vi "lin-log.vi"(4 "W In 1":dbl, 5 "W In 2":dbl, 6 "W In 3":dbl, 7 "W In 4":dbl) -> (0 "dBm Out 1":dbl, 1 "dBm Out 2":dbl, 2 "dBm Out 3":dbl, 3 "dBm Out 4":dbl)   [LabVIEW 2015]
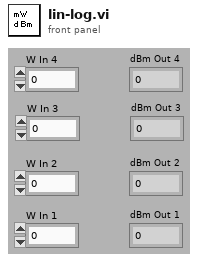
[diagram p1: front panel]
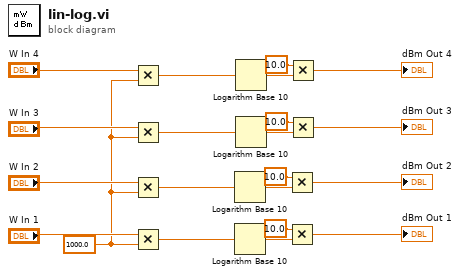
[diagram p0: block diagram]
diagram:
  w1 = 1000.0 ("y")
  n1 = Multiply(x="W In 4", y=w1) -> (x*y=w6:dbl)
  n2 = Multiply(x="W In 3", y=w1) -> (x*y=w7:dbl)
  n3 = Multiply(x="W In 2", y=w1) -> (x*y=w8:dbl)
  n4 = Multiply(x="W In 1", y=w1) -> (x*y=w9:dbl)
  n5 = Logarithm Base 10(1:w8) -> (0:w18:dbl)
  n6 = Logarithm Base 10(1:w9) -> (0:w20:dbl)
  n7 = Logarithm Base 10(1:w6) -> (0:w14:dbl)
  n8 = Logarithm Base 10(1:w7) -> (0:w16:dbl)
  n9 = Multiply(x=10.0, y=w18) -> (x*y=→"dBm Out 2":dbl)
  n10 = Multiply(x=10.0, y=w20) -> (x*y=→"dBm Out 1":dbl)
  n11 = Multiply(x=10.0, y=w14) -> (x*y=→"dBm Out 4":dbl)
  n12 = Multiply(x=10.0, y=w16) -> (x*y=→"dBm Out 3":dbl)
